vi "BotSpeak_IPAddr.vi"() -> (0 "response":string="Test")   [LabVIEW 2014]
doc: "Returns the IP address of the associated RIO as \"response\"."
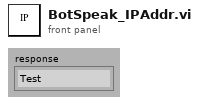
[diagram p1: front panel]
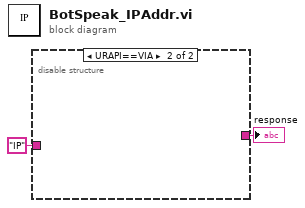
[diagram p0: block diagram]
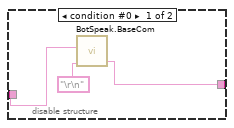
[diagram p2: hidden frame]
diagram:
  n1 = disable-structure shown="URAPI==VIA" {
    disable-tunnel: [w4 _] -> w2
    disable-tunnel: "IP" ("command") -> [w3 _]
    frame condition #0 {
      n2 = call <userlib>:"BotSpeak.BaseCom.vi"("Termination"="\r\n", "command"=w3) -> ("response"=w4:string)  [unwired: 3 in, 1 out]
    }
    frame condition #1 (active) {
    }
  }
  "response" <- w2
